vi "defectiveSpareParts.vi"(0 "reference in":refnum<class "excelFile.lvclass">, 2 "data":string[][](array[string]), 3 "O2 exp date":string, 5 "error in (no error)":errorcluster) -> (14 "reference out":refnum<class "excelFile.lvclass">, 19 "error out":errorcluster)   [LabVIEW 2016, in "excelFile.lvclass"]
uses:
  excelFile.lvclass
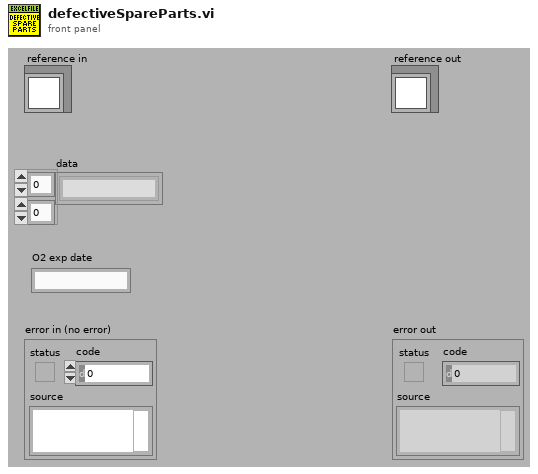
[diagram p1: front panel]
types:
  T1 = typedef "excelFile.lvclass/ObjectAttributesRef.ctl" = refnum<data-value>
  T2 = typedef "excelFile.lvclass/ObjectAttributes.ctl" = cluster{"MyAttribute":dbl, "path":string, "Refnum Excel":cluster{"Excel._Application":refnum<k7>, "Workbooks":refnum<k7>, "Open":refnum<k7>}, "data":string[][][], "save":bool, "fileType":T3, "rowsColor":u32[], "python_ref":refnum<class "python.lvclass">, "items_rows":i32[], "excel_range":i32[][], "TSR":cluster{"number":string, "TSR_path":path, "service_path":path, "email_to":string}, "excel_already_opened?":bool, "file_already_opened?":bool, "excel_protected_opened?":bool, "Refnum Cluster Worksheets":cluster{"Excel._Application":refnum<k7>, "Workbooks":refnum<k7>, "Open":refnum<k7>, "Worksheets":refnum<k7>, "Excel._Worksheet":refnum<k7>}, "#_rows_defective":i32, "#_rows_spare":i32}
  T3 = typedef "excelFile.lvclass/fileType.ctl" = enum16{"devices", "items", "partsTracking", "TSR"}
  T4 = cluster{"Excel._Application":refnum<k7>, "Workbooks":refnum<k7>, "Open":refnum<k7>, "Worksheets":refnum<k7>, "Excel._Worksheet":refnum<k7>}
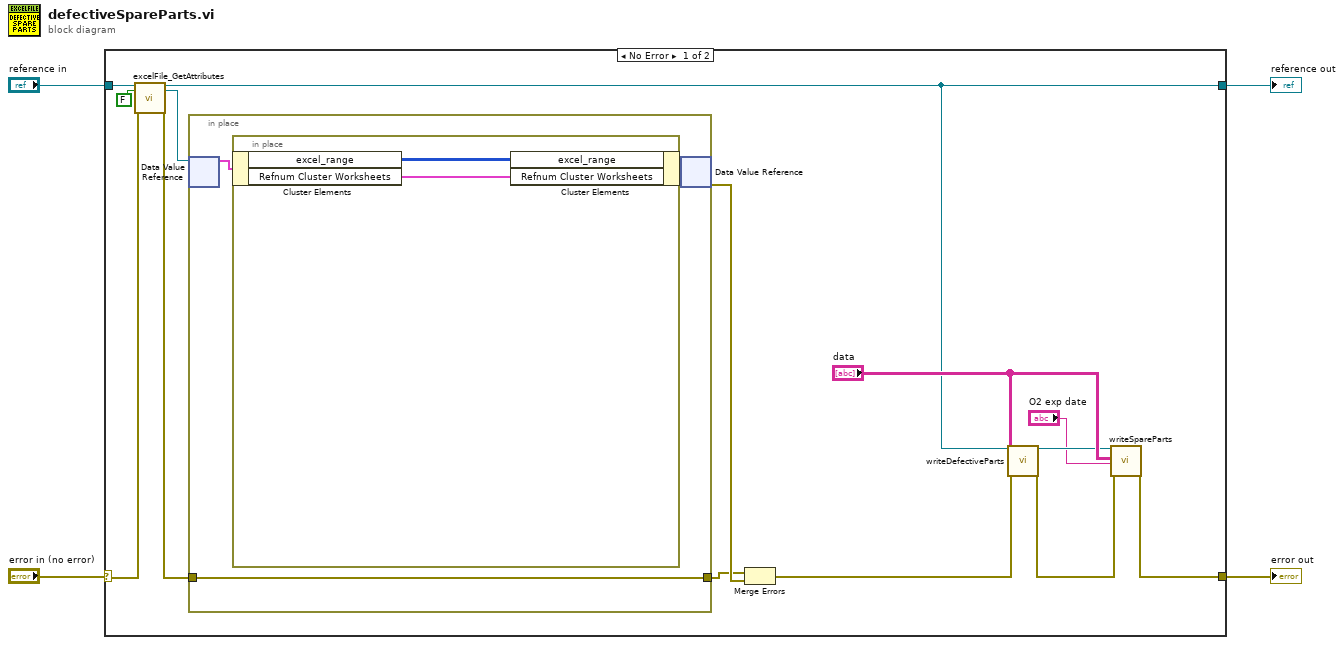
[diagram p0: block diagram]
diagram:
  n1 = case shown="No Error" "error in (no error)" {
    selector: "error in (no error)" -> [w14 w25]
    tunnel: [w6 w25] -> w3
    tunnel: [w9 w24] -> w1
    tunnel: "reference in" -> [w16 w24]
    frame No Error {
      n2 = call "excelFile_GetAttributes.vi"("reference in"=w16, "return data? (T)"=FALSE, "error in (no error)"=w14) -> ("reference out"=w9:refnum<class "excelFile.lvclass">, "attributes ref"=w12:T1, "error out"=w13:errorcluster)  [unwired: 13 in, 1 out]
      n3 = in-place {
        in-place-border: w13 -> [w19]
        in-place-border: [w19] -> w17
        n4 = in-place-dvr #1(w12) -> (w20:T2)  [unwired: 1 out]
        n5 = in-place {
          n6 = in-place-cluster #2(w20) -> ("excel_range"=w23:i32[][], "Refnum Cluster Worksheets"=w22:T4)
          n7 = in-place-cluster #2("excel_range"=w23, "Refnum Cluster Worksheets"=w22) -> (w21:T2)
        }
        n8 = in-place-dvr #1(w21) -> (w18:errorcluster)  [unwired: 1 out]
      }
      n9 = Merge Errors(w17, w18) -> (w8:errorcluster)
      n10 = call "writeDefectiveParts.vi"("reference in"=w9, "data"="data", "error in (no error)"=w8) -> ("reference out"=w10:refnum<class "excelFile.lvclass">, "error out"=w7:errorcluster)  [unwired: 15 in]
      n11 = call "writeSpareParts.vi"("reference in"=w10, "data"="data", "O2 exp date"="O2 exp date", "error in (no error)"=w7) -> ("error out"=w6:errorcluster)  [unwired: 14 in, 1 out]
    }
    frame Error {
    }
  }
  "error out" <- w3
  "reference out" <- w1
